vi "csv_control _02.vi"() -> ()   [LabVIEW 2024]
panel:
  in  "Test_Value":dbl
  in  "Test_ID":string
  in  "SN":string
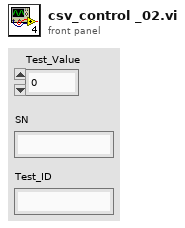
[diagram p1: front panel]
types:
  T1 = enum16{"open", "replace", "create", "open or create", "replace or create", "replace or create with confirmation"}
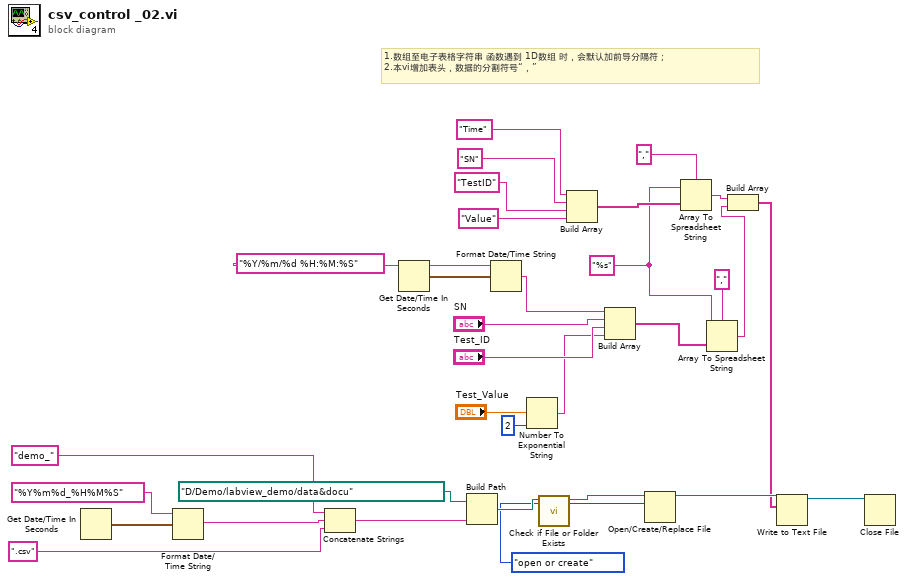
[diagram p0: block diagram]
diagram:
  w5 = "%s" ("格式字符串")
  # "1.数组至电子表格字符串 函数遇到 1D数组 时，会默认加前导分隔符；\n2.本vi增加表头，数据的分割符号“，”"
  n1 = Get Date/Time In Seconds() -> (seconds since 1Jan1904=w15:timestamp)
  n2 = Format Date/Time String(time format string (%c)="%Y%m%d_%H%M%S" ("时间格式字符串(%c)"), seconds (now)=w15) -> (date/time string=w13:string)  [unwired: 1 in]
  n3 = Concatenate Strings("demo_" ("字符串"), w13, ".csv" ("字符串")) -> (w17:string)
  n4 = Get Date/Time In Seconds() -> (seconds since 1Jan1904=w26:timestamp)
  n5 = Build Path(base path=path "D:/Demo/labview_demo/data&docu" ("基路径"), name or relative path=w17) -> (appended path=w32:path)
  n6 = Format Date/Time String(time format string (%c)="%Y/%m/%d %H:%M:%S" ("时间格式字符串(%c)"), seconds (now)=w26) -> (date/time string=w12:string)  [unwired: 1 in]
  n7 = Number To Exponential String(number="Test_Value", precision (6)=i16 2 ("精度(6)")) -> (E-format string=w27:string)  [unwired: 2 in]
  n8 = call <vilib>:"Check if File or Folder Exists.vi"("path"=w32) -> ("dup path"=w31:path)  [unwired: 8 in, 2 out]
  n9 = Build Array("Time" ("元素"), "SN" ("元素"), "TestID" ("元素"), "Value" ("元素")) -> (w6:string[])
  n10 = Build Array(w12, "SN", "Test_ID", w27) -> (w24:string[])
  n11 = Open/Create/Replace File(file path (use dialog)=w31, operation (0:open)=T1."open or create" ("操作(0:open)")) -> (refnum out=w22:refnum<file>)  [unwired: 4 in, 2 out]
  n12 = Array To Spreadsheet String(delimiter (Tab)="," ("分隔符(Tab)"), array=w6, 3:w5) -> (spreadsheet string=w3:string)
  n13 = Array To Spreadsheet String(delimiter (Tab)="," ("分隔符(Tab)"), array=w24, 3:w5) -> (spreadsheet string=w2:string)
  n14 = Build Array(w3, w2) -> (w1:string[])
  n15 = Write to Text File(file (use dialog)=w22, text=w1) -> (refnum out=w21:refnum<file>)  [unwired: 2 in, 2 out]
  n16 = Close File(refnum=w21) -> ()  [unwired: 1 in, 2 out]
